vi "Initialize DG BME.vi"(8 "error in (no error)":errorcluster, 9 "DG Number":i32, 10 "Slot Number":i32, 11 "DG Product":i32(ring) items=["SRS_DG135"=1, "BME_DP01"=2, "BME_G02V3"=3, "BME_SG02V4"=4, "BME_G04"=5, "BME_G02V1"=6, "BME_G02V2"=7, "BME_SG02V1"=8, "BME_SG02V2"=9, "BME_SG02V3"=10, "BME_G03V1"=11, "BME_G03V2"=12, "BME_SG02V5"=13, "BME_G03V3"=14, "BME_G03V4"=15, "BME_SG02V6"=16, "BME_G03V5"=17, "BME_G05V1"=18, "BME_G05V2"=19, "BME_G05V3"=20, "BME_SG02V7"=21, "BME_SG02P1"=31, "BME_G03P1"=32, "BME_G05P1"=33, "BME_SG02P2"=34, "BME_G03P2"=35, "BME_SG02P3"=36, "BME_SG05P1"=37, "BME_G05P2"=38, "BME_SG05P2"=39, "BME_G05P3"=40, "BME_SG02P4"=41, "BME_SG02P5"=42, "BME_SG05P3"=43, "BME_SG08P1"=44]) -> (0 "error out":errorcluster)   [LabVIEW 2009]
doc: "long Initialize_DG_BME(long base, long Product, long DG_Number);"
uses:
  DelayGenerator.dll
panel:
  # "NOTICE -- YOU MUST LEAVE THIS NOTICE IN PLACE.  PER THE TERMS OF THE LICENSE BELOW, YOU MAY SUBLICENSE THIS SOFTWARE \nIN ANY WAY THAT DOES NOT CONFLICT WITH THIS LICENSE.\n\n### BSD License (http://www.opensource.org/licenses/bsd-license.php) Begin ###\n \nCopyright (c) 2011, Applied Energetics, http://www.appliedenergetics.com,\n                               Richard Schwerdtfeger, <rschwerdtfeger@appliedenergetics.com>\n\nAll rights reserved.\n\nRedistribution and use in source and binary forms, with or without modification, are permitted provided that the \nfollowing conditions are met:\n\n    * Redistributions of source code must retain the above copyright notice, this list of conditions and the following disclaimer.\n    * Redistributions in binary form must reproduce the above copyright notice, this list of conditions and the following disclaimer \n       in the documentation and/or other materials provided with the distribution.\n    * Neither the name of Richard Schwerdtfeger, Applied Energetics, Inc., nor the names of its contributors may be used to \n       endorse or promote products derived from this software without specific prior written permission.\n\nTHIS SOFTWARE IS PROVIDED BY THE COPYRIGHT HOLDERS AND CONTRIBUTORS \"AS IS\" AND ANY EXPRESS OR IMPLIED WARRANTIES, \nINCLUDING, BUT NOT LIMITED TO, THE IMPLIED WARRANTIES OF MERCHANTABILITY AND FITNESS FOR A PARTICULAR PURPOSE ARE \nDISCLAIMED. IN NO EVENT SHALL THE COPYRIGHT OWNER OR CONTRIBUTORS BE LIABLE FOR ANY DIRECT, INDIRECT, INCIDENTAL,\n SPECIAL, EXEMPLARY, OR CONSEQUENTIAL DAMAGES (INCLUDING, BUT NOT LIMITED TO, PROCUREMENT OF SUBSTITUTE GOODS OR \nSERVICES; LOSS OF USE, DATA, OR PROFITS; OR BUSINESS INTERRUPTION) HOWEVER CAUSED AND ON ANY THEORY OF LIABILITY, \nWHETHER IN CONTRACT, STRICT LIABILITY, OR TORT (INCLUDING NEGLIGENCE OR OTHERWISE) ARISING IN ANY WAY OUT OF THE USE \nOF THIS SOFTWARE, EVEN IF ADVISED OF THE POSSIBILITY OF SUCH DAMAGE.\n\n### BSD License End ###"
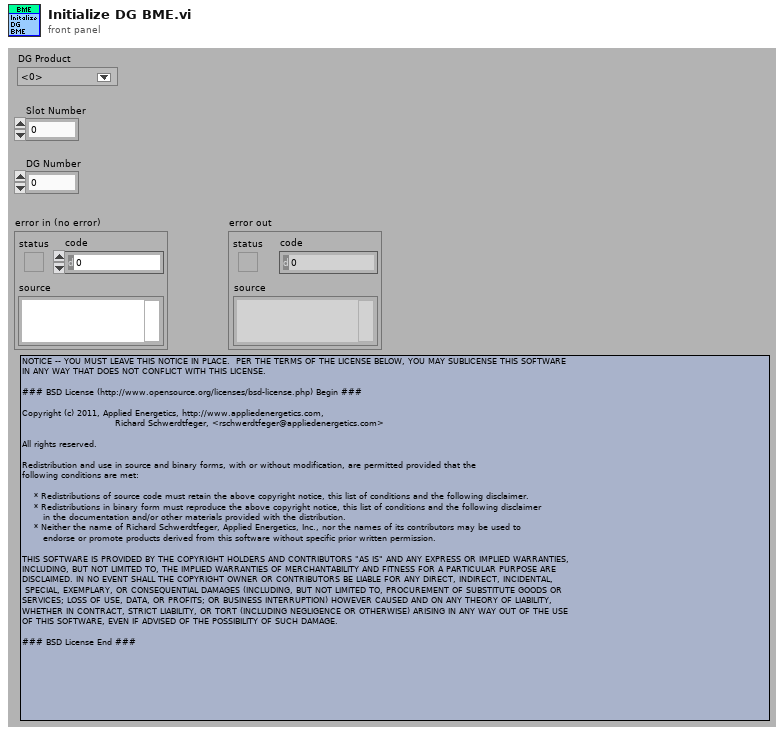
[diagram p1: front panel]
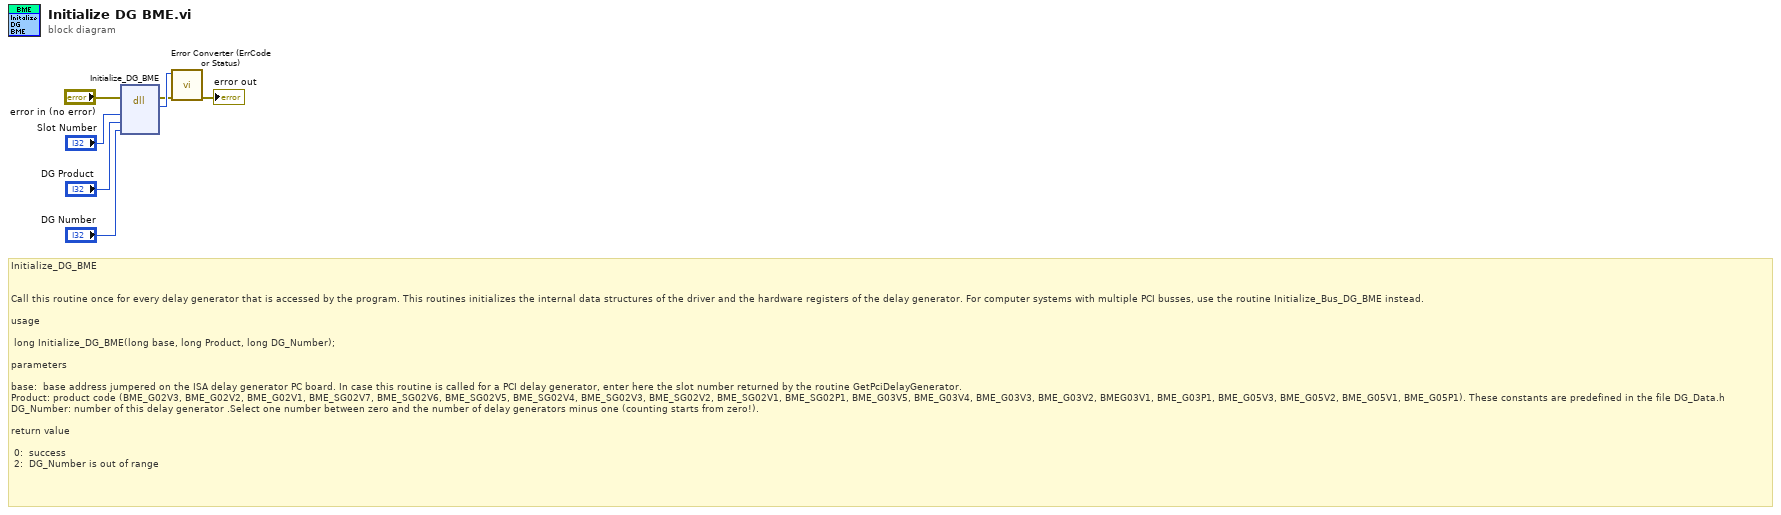
[diagram p0: block diagram]
diagram:
  # "Initialize_DG_BME\n\n\nCall this routine once for every delay generator that is accessed by the program. This routines initializes the internal data structures of the driver and the hardware registers of the delay generator. For computer systems with multiple PCI busses, use the routine Initialize_Bus_DG_BME instead.\n\nusage\n\n\tlong Initialize_DG_BME(long base, long Product, long DG_Number);\n\nparameters\n\nbase:\t\tbase address jumpered on the ISA delay generator PC board. In case this routine is called for a PCI delay generator, enter here the slot number returned by the routine GetPciDelayGenerator.\nProduct:\tproduct code (BME_G02V3, BME_G02V2, BME_G02V1, BME_SG02V7, BME_SG02V6, BME_SG02V5, BME_SG02V4, BME_SG02V3, BME_SG02V2, BME_SG02V1, BME_SG02P1, BME_G03V5, BME_G03V4, BME_G03V3, BME_G03V2, BMEG03V1, BME_G03P1, BME_G05V3, BME_G05V2, BME_G05V1, BME_G05P1). These constants are predefined in the file DG_Data.h\nDG_Number:\tnumber of this delay generator .Select one number between zero and the number of delay generators minus one (counting starts from zero!).\n\nreturn value\n\n\t0:  success\n\t2:  DG_Number is out of range"
  n1 = dll-call lib="C:/Dokumente und Einstellungen/A2.5/Desktop/BME_SW Stand 201203-26/LabView_SG08p/BME Delay Generator/DelayGenerator.*" fn="Initialize_DG_BME"(error in="error in (no error)", "Slot"="Slot Number", "Product"="DG Product", "DG_Number"="DG Number") -> (error out=w2:errorcluster, "return type"=w7:i32)  [unwired: 5 in, 1 out]
  n2 = call "Error Converter (ErrCode or Status).vi"("error in (no error)"=w2, "error code"=w7) -> ("error out"=→"error out":errorcluster)  [unwired: 9 out]
